vi "Polling.vi"(8 "error in (no error)":errorcluster, 11 "Node Ptr":T1 format="%.0x") -> (0 "error out":errorcluster)   [LabVIEW 2019, in "Diagnostics Addon System Explorer.lvlib"]
uses:
  Diagnostics Addon System Explorer.lvlib
  <vilib>/NI VeriStand/Custom Device API/Custom Device API.lvlib
  Types/FG.Action.ctl
  <vilib>/NI VeriStand/Custom Device API/Custom Device Item Ref.ctl
panel:
  in  "SHDocVw.IWebBrowser":refnum<k7>(container)
  in  "Collection":i32(listbox) caption="Items"
  in  "Description":string
  out "Name":string
  in  "Header":cluster{"Section Name":string}={"Section Name"="Custom Device Item Settings"}
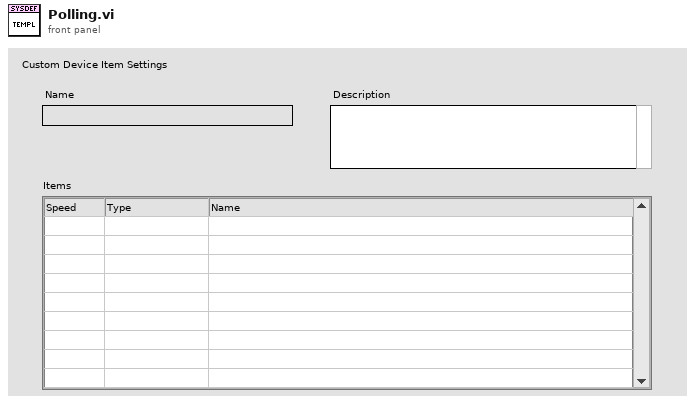
[diagram p1: front panel]
types:
  T1 = typedef "Custom Device API.lvlib/Custom Device Item Ref.ctl" = u64
  T2 = typedef "Diagnostics Addon System Explorer.lvlib/FG.Action.ctl" = enum16{"Get", "Set"}
  T3 = typedef "Custom Device API.lvlib/Custom Device Item Info.ctl" = cluster{"Name":string, "Is Channel":bool, "GUID":string, "Is Waveform":bool}
  T4 = typedef "Diagnostics Addon System Explorer.lvlib/Poll.LinkedNode.ctl" = cluster{"Node ID":u64}
  T5 = typedef "Custom Device API.lvlib/Custom Device Commands.ctl" = enum16{"Default", "Item renamed", "Shutdown", "Dynamic button pressed"}
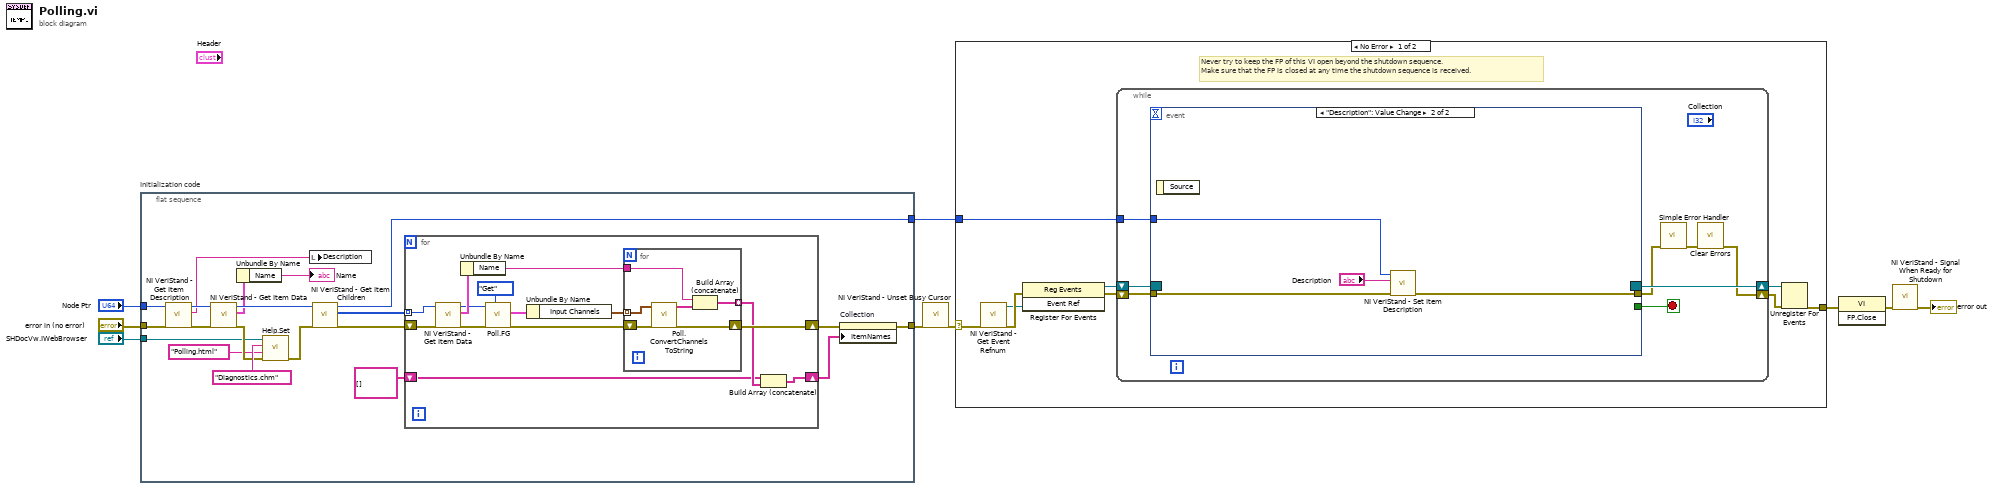
[diagram p0: block diagram]
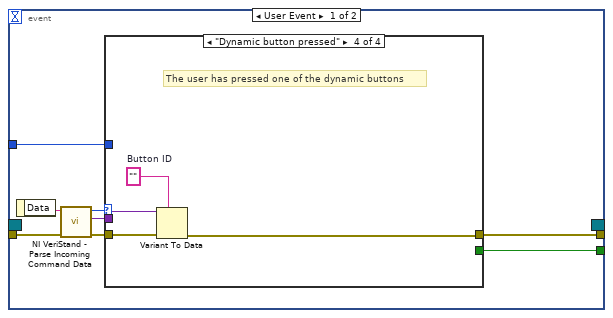
[diagram p2: hidden frame]
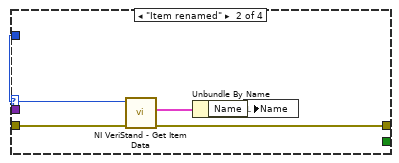
[diagram p4: hidden frame]
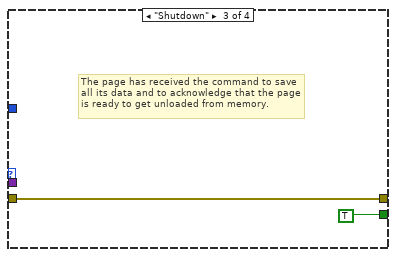
[diagram p5: hidden frame]
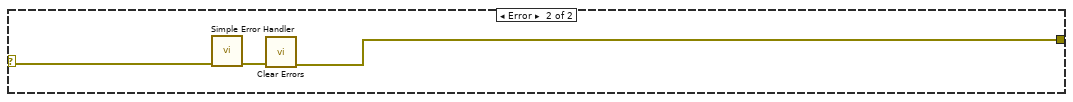
[diagram p6: hidden frame]
diagram:
  n1 = flat-sequence "Initialization code" {
    tunnel: "error in (no error)" -> [w13]
    tunnel: [w18] -> w6
    tunnel: [w20] -> w3
    tunnel: "Node Ptr" -> [w23]
    tunnel: "SHDocVw.IWebBrowser" -> [w14]
    frame #0 {
      n2 = call <vilib>:"NI VeriStand - Get Item Description.vi"("error in (no error)"=w13, "Item Ref in"=w23) -> ("error out"=w26:errorcluster, "Description"=w27:string, "Item Ref out"=w28:T1)  [unwired: 7 out]
      n3 = call <vilib>:"NI VeriStand - Get Item Data.vi"("error in (no error)"=w26, "Item Ref in"=w28) -> ("error out"=w16:errorcluster, "Item Info"=w25:T3, "Item Ref out"=w29:T1)  [unwired: 7 out]
      n4 = Unbundle By Name(w25) -> ("Name"=→"Name":string)
      n5 = call "Help.Set.vi"("error in (no error)"=w16, "HTML File"="Polling.html", "Main CHM File"="Diagnostics.chm", "SHDocVw.IWebBrowser2"=w14) -> ("error out"=w15:errorcluster)  [unwired: 7 in]
      n6 = local write "Description"(w27) -> ()
      n7 = call <vilib>:"NI VeriStand - Get Item Children.vi"("error in (no error)"=w15, "Item Ref in"=w29) -> ("error out"=w22:errorcluster, "Child Refs"=w21:T1[], "Item Ref out"=w20:T1)  [unwired: 6 in, 1 out]
      n8 = for {
        shift-right: [w34] -> w19
        shift-left: w22 -> [w42]
        tunnel: w21 -> [w41] mode=indexing
        shift-right: [w31] -> w11
        shift-left: string[][] [] -> [w30]
        n9 = call <vilib>:"NI VeriStand - Get Item Data.vi"("error in (no error)"=w42, "Item Ref in"=w41) -> ("error out"=w37:errorcluster, "Item Info"=w43:T3, "Item Ref out"=w36:T1)  [unwired: 7 out]
        n10 = Unbundle By Name(w43) -> ("Name"=w33:string)
        n11 = call "Poll.FG.vi"("Action"=FG.Action."Get", "error in"=w37, "Parent Ref"=w36) -> ("error out"=w35:errorcluster, "Selected Channels out"=w38:cluster{"Input Channels":T4[]})  [unwired: 6 in, 1 out]
        n12 = Unbundle By Name(w38) -> ("Input Channels"=w39:T4[])
        n13 = for {
          shift-right: [w47] -> w34
          shift-left: w35 -> [w49]
          tunnel: w39 -> [w48] mode=indexing
          tunnel: [w44] -> w32 mode=indexing
          tunnel: w33 -> [w46]
          n14 = call "Poll.ConvertChannelsToString.vi"("error in (no error)"=w49, "MonitoredChannelSettings"=w48) -> ("error out"=w47:errorcluster, "Array"=w45:string[])  [unwired: 8 in]
          n15 = Build Array (concatenate)(w46, w45) -> (w44:string[])
        }
        n16 = Build Array (concatenate)(w30, w32) -> (w31:string[][])
      }
      n17 = property on="Collection" class="MCListbox (strict)"(error in=w19, "ItemNames"=w11) -> (error out=w18:errorcluster)  [unwired: 1 in, 1 out]
    }
  }
  n18 = call <vilib>:"NI VeriStand - Unset Busy Cursor.vi"("error in (no error)"=w6) -> ("error out"=w5:errorcluster)  [unwired: 10 out]
  n19 = case shown="No Error" w5 {
    selector: w5 -> [w50 w93]
    tunnel: [w55 w91] -> w9
    tunnel: w3 -> [w51 _]
    frame No Error {
      # "Never try to keep the FP of this VI open beyond the shutdown sequence.\nMake sure that the FP is closed at any time the shutdown sequence is received."
      n20 = call <vilib>:"NI VeriStand - Get Event Refnum.vi"("error in (no error)"=w50) -> ("error out"=w58:errorcluster, "Event Ref"=w54:refnum<user-event>)  [unwired: 9 out]
      n21 = register-events(error in=w58, w54) -> (reference out=w52:refnum<event-registration>, error out=w53:errorcluster)  [unwired: 1 in]
      n22 = while {
        tunnel: w51 -> [w62]
        shift-right: [w59] -> w56
        shift-left: w53 -> [w65]
        shift-right: [w66] -> w57
        shift-left: w52 -> [w64]
        stop <- w63 stop-if-true
        n23 = event shown="[1] \"Description\": Value Change" {
          selector: w64 -> [_ _]
          dyn-events: [_ _] -> w66
          timeout: _ -> [_ _]
          tunnel: w65 -> [w74 w89]
          tunnel: [w70 _] -> w63
          tunnel: [w69 w88] -> w61
          tunnel: w62 -> [w68 w90]
          event User Event {
            n24 = event-data() -> ("Data"=w73:string)  [unwired: 1 out]
            n25 = call <vilib>:"NI VeriStand - Parse Incoming Command Data.vi"("error in (no error)"=w74, "Incoming data"=w73) -> ("error out"=w72:errorcluster, "Outgoing data"=w67:variant, "Action"=w71:T5)  [unwired: 7 out]
            n26 = case shown="\"Dynamic button pressed\"" w71 {
              tunnel: w72 -> [w75 w80 w81 w86]
              tunnel: [_ _ TRUE _] -> w70
              tunnel: [w75 w77 w81 w83] -> w69
              tunnel: w68 -> [_ w79 _ _]
              tunnel: w67 -> [_ _ _ w85]
              frame "Default", Default {
              }
              frame "Item renamed" {
                n27 = call <vilib>:"NI VeriStand - Get Item Data.vi"("error in (no error)"=w80, "Item Ref in"=w79) -> ("error out"=w77:errorcluster, "Item Info"=w78:T3)  [unwired: 8 out]
                n28 = Unbundle By Name(w78) -> ("Name"=w76:string)
                n29 = local write "Name"(w76) -> ()
              }
              frame "Shutdown" {
                # "The page has received the command to save all its data and to acknowledge that the page is ready to get unloaded from memory."
              }
              frame "Dynamic button pressed" {
                w84 = ""  # Button ID
                # "The user has pressed one of the dynamic buttons"
                n30 = Variant To Data(error in=w86, type=w84, Variant=w85) -> (error out=w83:errorcluster)  [unwired: 1 out]
              }
            }
          }
          event "Description": Value Change {
            n31 = event-data() -> ()  [unwired: 2 out]
            n32 = call <vilib>:"NI VeriStand - Set Item Description.vi"("error in (no error)"=w89, "Description"="Description", "Item Ref in"=w90) -> ("error out"=w88:errorcluster)  [unwired: 8 out]
          }
        }
        n33 = call <vilib>:"Simple Error Handler.vi"("error in (no error)"=w61) -> ("error out"=w60:errorcluster)  [unwired: 1 in, 7 out]
        n34 = call <vilib>:"Clear Errors.vi"("error in (no error)"=w60) -> ("error out"=w59:errorcluster)  [unwired: 1 in, 5 out]
      }
      n35 = Unregister For Events(event registration refnum=w57, error in=w56) -> (error out=w55:errorcluster)
    }
    frame Error {
      n36 = call <vilib>:"Simple Error Handler.vi"("error in (no error)"=w93) -> ("error out"=w92:errorcluster)  [unwired: 1 in, 7 out]
      n37 = call <vilib>:"Clear Errors.vi"("error in (no error)"=w92) -> ("error out"=w91:errorcluster)  [unwired: 1 in, 5 out]
    }
  }
  n38 = invoke class="VI" method="FP.Close"(error in=w9) -> (error out=w8:errorcluster)  [unwired: 2 in, 2 out]
  n39 = call <vilib>:"NI VeriStand - Signal When Ready for Shutdown.vi"("error in (no error)"=w8) -> ("error out"=→"error out":errorcluster)  [unwired: 10 out]
